vi "Query Output.vi"(8 "error in (no error)":errorcluster, 11 "VISA resource name":refnum<visa-resource-name>) -> (0 "error out":errorcluster, 2 "Output On?":bool, 3 "VISA resource name out":refnum<visa-resource-name>)   [LabVIEW 2023, in "Agilent PSG MXG Series.lvlib"]
uses:
  Agilent PSG MXG Series.lvlib
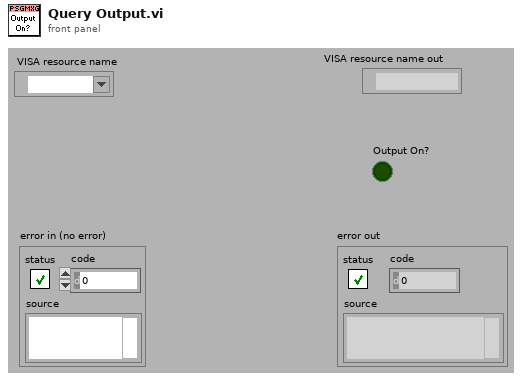
[diagram p1: front panel]
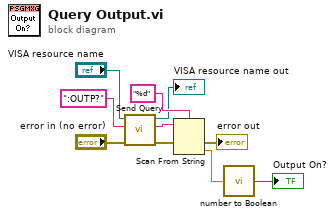
[diagram p0: block diagram]
diagram:
  n1 = call "Send Query.vi"("error in (no error)"="error in (no error)", "write buffer"=":OUTP?", "VISA resource name"="VISA resource name") -> ("error out"=w2:errorcluster, "read buffer"=w7:string, "VISA resource name out"=→"VISA resource name out":refnum<visa-resource-name>)  [unwired: 6 out]
  n2 = Scan From String(format string="%d", input string=w7, error in=w2) -> (error out=→"error out":errorcluster, output 1=w4:dbl)  [unwired: 1 in, 3 out]
  n3 = call "number to Boolean.vi"("Numeric"=w4) -> ("Boolean"=→"Output On?":bool)
